vi "Read IOPub.vi"(8 "error in (no error)":errorcluster, 11 "object in":refnum<class "JuPyter_Client.lvclass">) -> (0 "error out":errorcluster, 2 "data":string[](array[string]), 3 "object out":refnum<class "JuPyter_Client.lvclass">, 4 "timeout?":bool)   [LabVIEW 2018, in "JuPyter_Client.lvclass"]
doc: "Read data from the IOPub socket"
uses:
  JuPyter_Client.lvclass
  JuPyter_Client.lvclass/JuPyter_Client.ctl
  <vilib>/addons/zeromq/zeromq.lvlib
  <vilib>/addons/zeromq/zmq_socket.lvclass
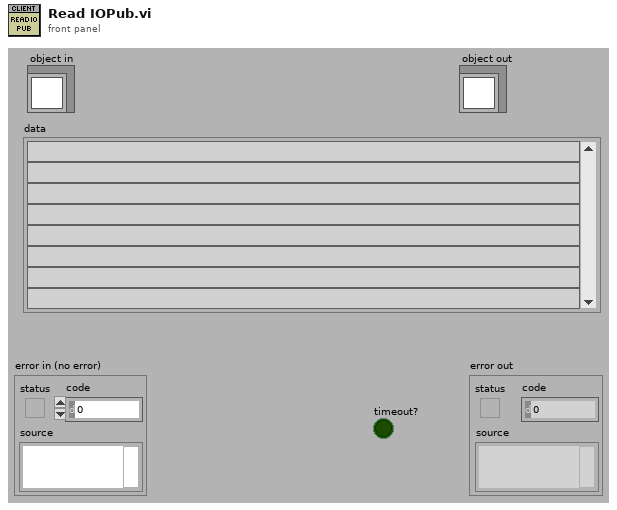
[diagram p1: front panel]
types:
  T1 = typedef "zeromq.lvlib/error_type.ctl" = enum16{"No Error", "EUNKNOWN", "ENOTSUP", "EPROTONOSUPPORT", "ENOBUFS", "ENETDOWN", "EADDRINUSE", "EADDRNOTAVAIL", "ECONNREFUSED", "EINPROGRESS", "ENOTSOCK", "EMSGSIZE", "EAFNOSUPPORT", "ENETUNREACH", "ECONNABORT", "ECONNRESET", "ENOTCONN", "ETIMEDOUT", "EHOSTUNREACH", "ENETRESET", "EBUSY", "EINVAL", "ENODEV", "EFAULT", "EINTR", "ENOENT", "ENOMEM", "EAGAIN", "EMFILE", "EFSM", "ENOCOMPATPROTO", "ETERM", "EMTHREAD", "Invalid"}
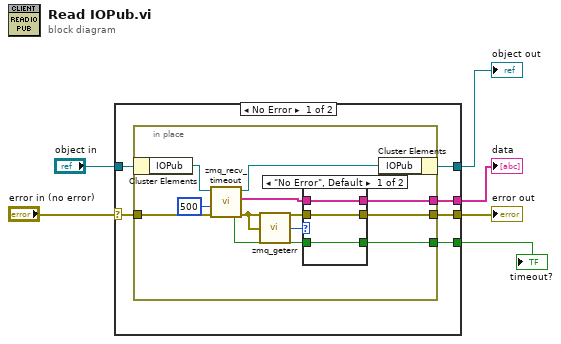
[diagram p0: block diagram]
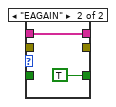
[diagram p2: hidden frame]
diagram:
  n1 = case shown="No Error" "error in (no error)" {
    selector: "error in (no error)" -> [w10 w30]
    tunnel: [w9 w30] -> w5
    tunnel: [w11 w29] -> w3
    tunnel: "object in" -> [w12 w29]
    tunnel: [w8 _] -> w1
    tunnel: [w7 _] -> w2
    frame No Error {
      n2 = in-place {
        in-place-border: w10 -> [w21]
        in-place-border: [w17] -> w9
        in-place-border: [w16] -> w8
        in-place-border: [w15] -> w7
        n3 = in-place-cluster #1(w12) -> ("IOPub"=w23:refnum<class "zmq_socket.lvclass">)
        n4 = call <vilib>:"zmq_recv_timeout.vi"("error in"=w21, "timeout (ms)"=u32 500, "socket in"=w23) -> ("error out"=w19:errorcluster, "timeout?"=w14:bool, "parts"=w18:string[], "socket out"=w22:refnum<class "zmq_socket.lvclass">)  [unwired: 1 in]
        n5 = call <vilib>:"zmq_geterr.vi"("error in"=w19) -> ("type"=w20:T1)
        n6 = case shown="\"No Error\", Default" w20 {
          tunnel: [w26 _] -> w17
          tunnel: w19 -> [w26 _]
          tunnel: [w25 w28] -> w16
          tunnel: w18 -> [w25 w28]
          tunnel: [w24 TRUE] -> w15
          tunnel: w14 -> [w24 _]
          frame "No Error", Default {
          }
          frame "EAGAIN" {
          }
        }
        n7 = in-place-cluster #1("IOPub"=w22) -> (w11:refnum<class "JuPyter_Client.lvclass">)
      }
    }
    frame Error {
    }
  }
  "error out" <- w5
  "object out" <- w3
  "data" <- w1
  "timeout?" <- w2
